vi "InitAction.vi"(6 "InstrumentName":string, 7 "VisaRessIn":refnum<visa-resource-name>, 8 "error in (no error)":errorcluster caption="entrée d'erreur (pas d'erreur)", 9 "FirstClassInst":bool, 10 "Function":string, 11 "GenData In":refnum<class "AppliedMotionDrive.lvclass"> caption="DNL_LabVIEW Object in") -> (0 "error out":errorcluster caption="sortie d'erreur", 3 "GenData Out":refnum<class "AppliedMotionDrive.lvclass"> caption="DNL_LabVIEW Object out")   [LabVIEW 2019, in "AppliedMotionDrive.lvclass"]
uses:
  AppliedMotionDrive.lvclass
  C:/Programmes Labview/LabscanV1A/DevicesClass/BaseDevice/BaseDevice.lvclass
  AppliedMotionDrive_Func.ctl
  AppliedMotionDrive.lvclass/AppliedMotionDrive.ctl
  <vilib>/Utility/error.llb/DialogType.ctl
panel:
  in  "DefaultDev_Func":T1
  out "VisaRessOut":refnum<visa-resource-name>
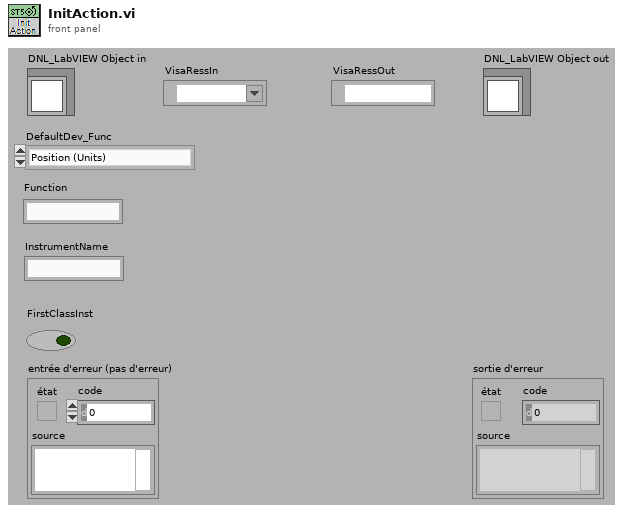
[diagram p1: front panel]
types:
  T1 = typedef "AppliedMotionDrive.lvclass/AppliedMotionDrive_Func.ctl" = enum16{"Position (Units)", "FilterWheel (Id)"}
  T2 = typedef "DialogType.ctl" = u16
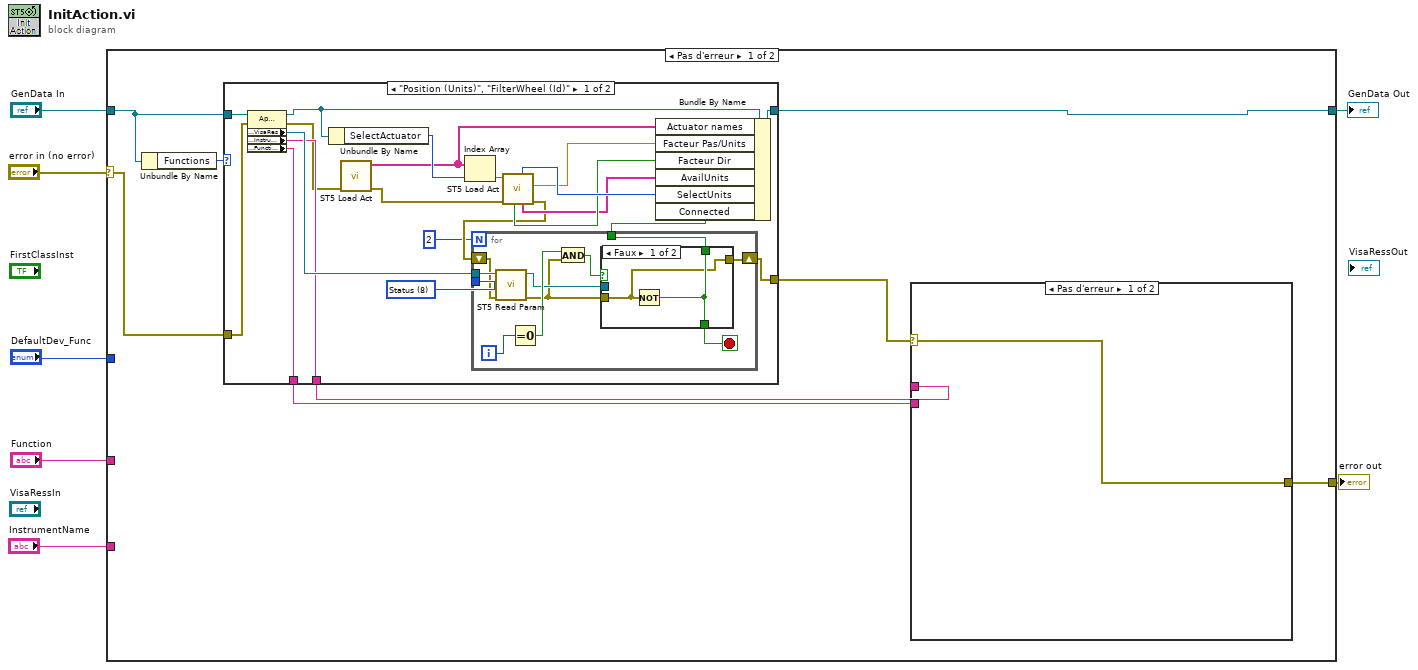
[diagram p0: block diagram]
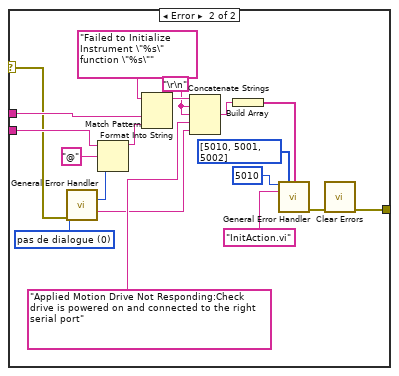
[diagram p2: hidden frame]
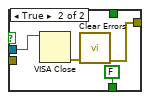
[diagram p3: hidden frame]
diagram:
  n1 = case shown="Pas d'erreur" "error in (no error)" {
    selector: "error in (no error)" -> [w13 w77]
    tunnel: [w11 w77] -> w6
    tunnel: "GenData In" -> [w14 w76]
    tunnel: [w9 w76] -> w4
    tunnel: "DefaultDev_Func" -> [_ _]
    tunnel: "Function" -> [_ _]
    tunnel: "InstrumentName" -> [_ _]
    frame No Error {
      n2 = Unbundle By Name(w14) -> ("Functions"=w15:T1)
      n3 = case shown="\"Position (Units)\", \"FilterWheel (Id)\"" w15 {
        tunnel: w14 -> [w56 w74]
        tunnel: w13 -> [w55 w75]
        tunnel: [w37 w75] -> w10
        tunnel: [w52 _] -> w12
        tunnel: [w50 w74] -> w9
        tunnel: [w51 _] -> w8
        frame "Position (Units)", "FilterWheel (Id)" {
          w53 = u16 8 items=["All", "Velocity", "Acceleration", "Deceleration", "Max Acceleration", "Position", "Step/Rev", "Alarm Code", "Status"] ("Parameters")
          n4 = property class="AppliedMotionDrive.lvclass"(reference=w56, error in=w55) -> (reference out=w49:refnum<class "AppliedMotionDrive.lvclass">, error out=w48:errorcluster, "Accessor:VisaRes"=w54:refnum<visa-resource-name>, "Accessor:InstrumentName"=w51:string, "Accessor:Function"=w52:string)
          n5 = Unbundle By Name(w49) -> ("SelectActuator"=w47:u8)
          n6 = call <userlib>:"ST5 Load Act .vi"("error in (no error)"=w48) -> ("error out"=w44:errorcluster, "Actuator names"=w46:string[])  [unwired: 3 in, 6 out]
          n7 = Index Array(array=w46, index=w47) -> (element=w45:string)
          n8 = call <userlib>:"ST5 Load Act .vi"("error in (no error)"=w44, "Actuator Settings"=w45) -> ("error out"=w39:errorcluster, "Facteur Pas"=w42:dbl, "Unit Strings"=w40:string[], "Units"=w43:u16, "Facteur Dir"=w41:bool)  [unwired: 2 in, 3 out]
          n9 = for {
            N: 2 -> [_]
            tunnel: w54 -> [w67]
            tunnel: w53 -> [w66]
            tunnel: [w64] -> w38
            shift-right: [w59] -> w37
            shift-left: w39 -> [w65]
            i -> [w62]
            stop <- w57 stop-if-true
            n10 = call <userlib>:"ST5 Read Param.vi"("error in (no error)"=w65, "Parameters"=w66, "Port COM"=w67) -> ("error out"=w58:errorcluster, "Port COM Out"=w60:refnum<visa-resource-name>)  [unwired: 2 in, 5 out]
            n11 = Equal To 0?(x=w62) -> (x = 0?=w61:bool)
            n12 = And(x=w61, y=w58) -> (x .and. y?=w63:bool)
            n13 = case shown="Faux" w63 {
              tunnel: [w69 _] -> w64
              tunnel: w60 -> [_ w73]
              tunnel: [w68 w71] -> w59
              tunnel: w58 -> [w68 _]
              tunnel: [w69 FALSE] -> w57
              frame False {
                n14 = Not(x=w68) -> (.not. x?=w69:bool)
              }
              frame True {
                n15 = VISA Close(VISA resource name=w73) -> (error out=w72:errorcluster)  [unwired: 1 in]
                n16 = call <vilib>:"Clear Errors.vi"("error in (no error)"=w72) -> ("error out"=w71:errorcluster)  [unwired: 5 in, 1 out]
              }
            }
          }
          n17 = Bundle By Name(cluster=w49, "Actuator names"=w46, "Facteur Pas/Units"=w42, "Facteur Dir"=w41, "AvailUnits"=w40, "SelectUnits"=w43, "Connected"=w38) -> (w50:refnum<class "AppliedMotionDrive.lvclass">)
        }
        frame Default {
        }
      }
      n18 = case shown="Pas d'erreur" w10 {
        selector: w10 -> [w16 w19]
        tunnel: [w16 w25] -> w11
        tunnel: w8 -> [_ w28]
        tunnel: w12 -> [_ w27]
        frame No Error {
        }
        frame Error {
          w18 = T2 0 items=["pas de dialogue", "Message OK", "Message continuer ou arrêter", "Message OK + mises en garde", "Arrêter/Continuer + mises en garde"] ("type of dialog (OK msg:1)")
          w21 = "\r\n"
          n19 = call <vilib>:"General Error Handler.vi"("type of dialog (OK msg:1)"=w18, "error in (no error)"=w19) -> ("code out"=w20:i32, "message"=w17:string)  [unwired: 9 in, 3 out]
          n20 = Match Pattern(string=w27, regular expression="@" ("chaîne"), offset (0)=w20) -> (before substring=w35:string)  [unwired: 3 out]
          n21 = Format Into String(format string="Failed to Initialize Instrument \"%s\" function \"%s\"" ("[error source] (\" \")"), w28, w35) -> (resulting string=w30:string)  [unwired: 2 in, 1 out]
          n22 = Concatenate Strings(w30, w21, w21, "Applied Motion Drive Not Responding:Check drive is powered on and connected to the right serial port", w17) -> (w24:string)
          n23 = Build Array(w24) -> (w23:string[])
          n24 = call <vilib>:"General Error Handler.vi"("[error code] (0)"=5010, "[user-defined codes]"=i32[] [5010, 5001, 5002], "[user-defined descriptions]"=w23, "[error source] (\" \")"="InitAction.vi" ("[error source] (\" \")")) -> ("error out"=w26:errorcluster)  [unwired: 7 in, 4 out]
          n25 = call <vilib>:"Clear Errors.vi"("error in (no error)"=w26) -> ("error out"=w25:errorcluster)  [unwired: 5 in, 1 out]
        }
      }
    }
    frame Error {
    }
  }
  "error out" <- w6
  "GenData Out" <- w4
